vi "User Input Handling.vi"(0 "Record?":bool, 1 "Get Tension":bool, 2 "Short":bool, 3 "Charge Time (s)":dbl, 4 "Short Wire Length (mm)":dbl, 5 "Long Wire Length (mm)":dbl, 6 "Sampling Time (s)":i32) -> (12 "Has measured?":bool=TRUE, 13 "Made Measurement?":bool, 14 "t < X ?":bool, 15 "DAQ":dbl, 16 "charging":bool, 17 "Elapsed time(s)":dbl caption="Elapsed Time (s)", 18 "Wire Length Out":dbl, 19 "Nth Measurement":i32)   [LabVIEW 2018]
uses:
  <vilib>/ptbypt/NI_PtbyPt.lvlib
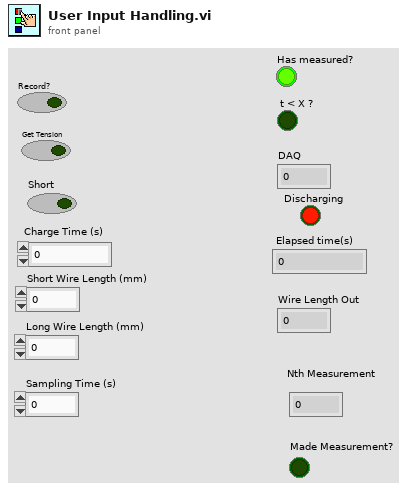
[diagram p1: front panel]
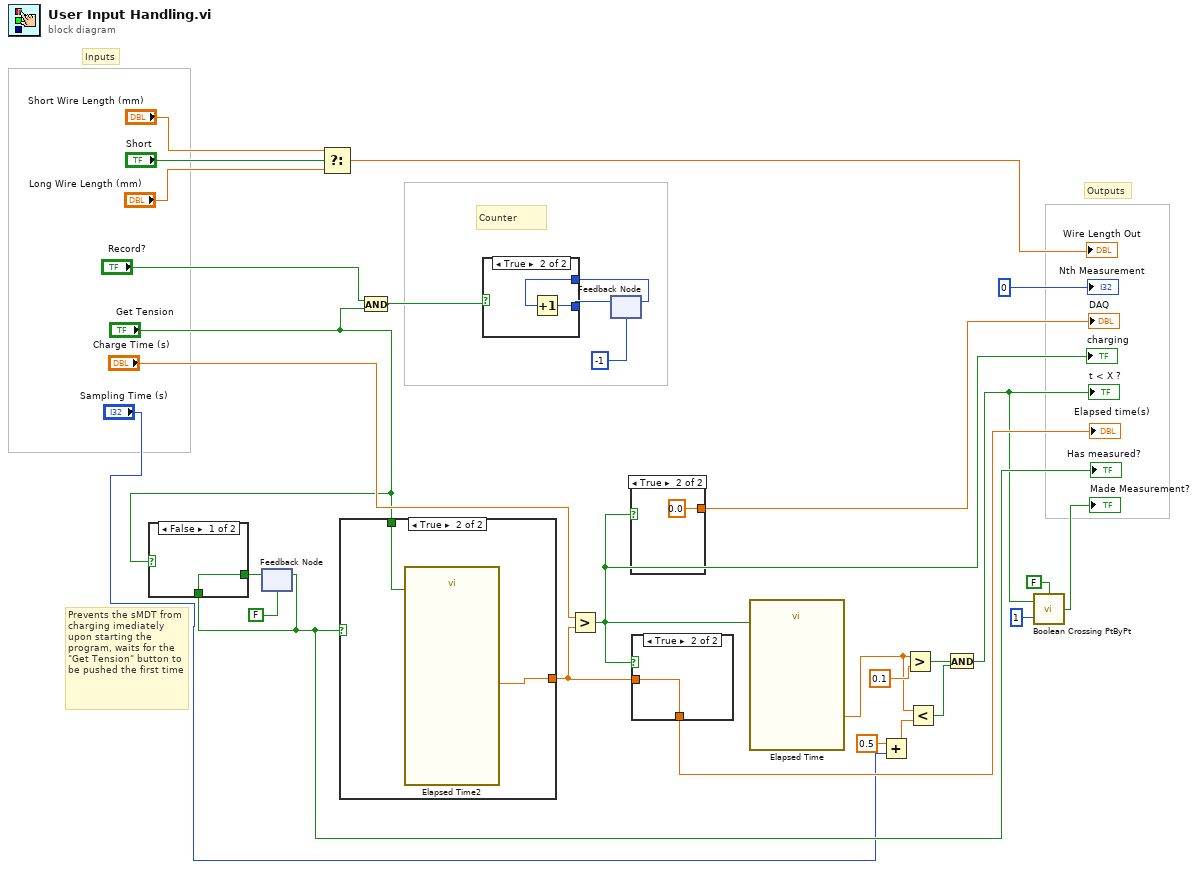
[diagram p0: block diagram]
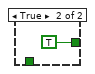
[diagram p3: hidden frame]
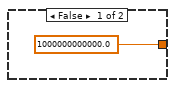
[diagram p4: hidden frame]
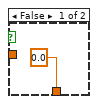
[diagram p5: hidden frame]
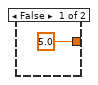
[diagram p6: hidden frame]
diagram:
  # "Prevents the sMDT from charging imediately upon starting the program, waits for the \"Get Tension\" button to be pushed the first time"
  # "Outputs"
  # "Inputs"
  # "Counter"
  n1 = feedback #1(FALSE) -> (w19:bool)
  "Has measured?" <- w19
  n2 = case shown="False" "Get Tension" {
    tunnel: [w31 TRUE] -> w22
    tunnel: w19 -> [w31 _]
    frame False {
    }
    frame True {
    }
  }
  n3 = feedback-in #1(w22) -> ()
  n4 = Select(t="Short Wire Length (mm)", s="Short", f="Long Wire Length (mm)") -> (s? t:f=→"Wire Length Out":dbl)
  n5 = case shown="True" w19 {
    tunnel: "Get Tension" -> [_ w35]
    tunnel: [1000000000000.0 w34] -> w20
    frame False {
    }
    frame True {
      n6 = call "Elapsed Time2"("Reset"=w35) -> ("Elapsed Time (s)"=w34:dbl)  [unwired: 11 in, 7 out]
    }
  }
  n7 = And(x="Record?", y="Get Tension") -> (x .and. y?=w4:bool)
  n8 = Greater?(x="Charge Time (s)", y=w20) -> (0:w23:bool)
  "charging" <- w23
  n9 = feedback #2(-1) -> (w5:i32)
  n10 = case shown="True" w4 {
    tunnel: [w36 w38] -> w6
    tunnel: w5 -> [w36 w37]
    frame False {
    }
    frame True {
      n11 = Increment(x=w37) -> (x+1=w38:i32)
    }
  }
  n12 = feedback-in #2(w6) -> ()
  n13 = case shown="True" w23 {
    tunnel: [5.0 0.0] -> w30
    frame False {
    }
    frame True {
    }
  }
  "DAQ" <- w30
  n14 = case shown="True" w23 {
    tunnel: w20 -> [_ w42]
    tunnel: [0.0 w42] -> w29
    frame False {
    }
    frame True {
    }
  }
  "Elapsed time(s)" <- w29
  n15 = call "Elapsed Time"("Reset"=w23) -> ("Elapsed Time (s)"=w24:dbl)  [unwired: 11 in, 7 out]
  n16 = Add(x=0.5, y="Sampling Time (s)") -> (x+y=w10:dbl)
  n17 = Greater?(x=w24, y=0.1) -> (0:w27:bool)
  n18 = Less?(x=w24, y=w10) -> (x < y?=w26:bool)
  n19 = And(x=w27, y=w26) -> (x .and. y?=w12:bool)
  "t < X ?" <- w12
  n20 = call <vilib>:"Boolean Crossing PtByPt.vi"("initialize"=FALSE, "direction"=1, "input"=w12) -> ("crossing"=→"Made Measurement?":bool)
  "Nth Measurement" <- 0 ("Nth Measurement")
